vi "Output.vi"(8 "error in (no error)":errorcluster, 11 "Pump Calibration Config in":T1={"Settings"={"Cycle Period"=500.0, "Ismatech"={"VISA resource name"="", "Simulated?"=TRUE, "Pump Number"=1.0, "Reverse?"=FALSE}, "Masterflex"={"VISA resource name"="", "Simulated?"=TRUE, "Pump Number"=1.0, "Reverse?"=FALSE}, "Bronkhorst M13 Settings"={"VISA resource name"="", "Simulated?"=TRUE, "Smoothing Steps"=1}, "PID 2 Parameters"={"Input Device"=enum."Default", "Output Device"=enum."Default"}, "Tacmina Settings"={"Analog DAQ Task"="", "Digital DAQ Task"=""}, "KNF SIMDOS Settings"={"VISA resource name"="", "Simulated?"=TRUE}, "VICI M50 Settings"={"VISA resource name"="", "Pump ID"="", "Pump Head Vol"=0.0, "Reverse?"=FALSE, "Simulated?"=TRUE}, "FLOM Settings"={"VISA resource name"="", "Simulated?"=TRUE, "Pump Number"=0.0}, "Calibration Limits"={"Minimum (ml/min)"=0.0, "Maximum (ml/min)"=0.0, "Steps"=0.0}, "SSI PR Settings"={"VISA resource name"="", "Simulated?"=FALSE}, "Ismatech 4308 Settings"={"VISA resource name"="", "Pump Number"=1, "Channel Number"=0, "Simulated?"=TRUE, "Reverse?"=FALSE}, "Bronkhorst M14 Settings"={"VISA resource name"="", "Simulated?"=FALSE, "Smoothing Steps"=1}}, "Flowmeter Output"=0.0, "Density"=0.0, "FL Temp"=0.0, "Speed %"=0.0, "File Refnum"=refnum, "Pump On?"=enum."Not Initialized"} {"Settings"."Bronkhorst M14 Settings"."Smoothing Steps" min=1 step=1; "Settings"."Ismatech 4308 Settings"."Channel Number" min=0 max=3; "Settings"."Ismatech 4308 Settings"."Pump Number" min=1; "Settings"."Bronkhorst M13 Settings"."Smoothing Steps" min=1 step=1; "Settings"."Masterflex"."Pump Number" min=1.0 max=20.0 step=1.0; "Settings"."Ismatech"."Pump Number" min=1.0 max=20.0 step=1.0}) -> (0 "error out":errorcluster, 3 "Pump Calibration Config Out":T1={"Settings"={"Cycle Period"=500.0, "Ismatech"={"VISA resource name"="", "Simulated?"=TRUE, "Pump Number"=1.0, "Reverse?"=FALSE}, "Masterflex"={"VISA resource name"="", "Simulated?"=TRUE, "Pump Number"=1.0, "Reverse?"=FALSE}, "Bronkhorst M13 Settings"={"VISA resource name"="", "Simulated?"=TRUE, "Smoothing Steps"=1}, "PID 2 Parameters"={"Input Device"=enum."Default", "Output Device"=enum."Default"}, "Tacmina Settings"={"Analog DAQ Task"="", "Digital DAQ Task"=""}, "KNF SIMDOS Settings"={"VISA resource name"="", "Simulated?"=TRUE}, "VICI M50 Settings"={"VISA resource name"="", "Pump ID"="", "Pump Head Vol"=0.0, "Reverse?"=FALSE, "Simulated?"=TRUE}, "FLOM Settings"={"VISA resource name"="", "Simulated?"=TRUE, "Pump Number"=0.0}, "Calibration Limits"={"Minimum (ml/min)"=0.0, "Maximum (ml/min)"=0.0, "Steps"=0.0}, "SSI PR Settings"={"VISA resource name"="", "Simulated?"=FALSE}, "Ismatech 4308 Settings"={"VISA resource name"="", "Pump Number"=1, "Channel Number"=0, "Simulated?"=TRUE, "Reverse?"=FALSE}, "Bronkhorst M14 Settings"={"VISA resource name"="", "Simulated?"=FALSE, "Smoothing Steps"=1}}, "Flowmeter Output"=0.0, "Density"=0.0, "FL Temp"=0.0, "Speed %"=0.0, "File Refnum"=refnum, "Pump On?"=enum."Not Initialized"} {"Settings"."Bronkhorst M14 Settings"."Smoothing Steps" min=1 step=1; "Settings"."Ismatech 4308 Settings"."Channel Number" min=0 max=3; "Settings"."Ismatech 4308 Settings"."Pump Number" min=1; "Settings"."Bronkhorst M13 Settings"."Smoothing Steps" min=1 step=1; "Settings"."Masterflex"."Pump Number" min=1.0 max=20.0 step=1.0; "Settings"."Ismatech"."Pump Number" min=1.0 max=20.0 step=1.0})   [LabVIEW 2018, in "Calibration.lvlib" / "Engine.lvlib"]
uses:
  Engine.lvlib
  Pump Calibration Config.ctl
  Pfizer Timed Seq/Software/Ismatec ISM 831C/Controls/Ismatech ISM831C Settings Cluster.ctl
  Pfizer Timed Seq/Software/Masterflex 7550-30/Controls/Settings Cluster.ctl
  Pfizer Timed Seq/Software/Bronkhorst M13 Flow Meter/Settings Cluster.ctl
  Pfizer Timed Seq/Software/Measure Instrument/PID Input Enum.ctl
  Pfizer Timed Seq/Software/Measure Instrument/PID 2 Output Enum.ctl
  Pfizer Timed Seq/Software/Tacmina QI/Tacmina QI DAQ Setting.ctl
  Pfizer Timed Seq/Software/KNF Pump/Settings Cluster plus SIMDOS.ctl
  Pfizer Timed Seq/Software/VICI M50 Party Mode/Settings Cluster.ctl
  Pfizer Timed Seq/Software/FLOM Pump/Settings Cluster.ctl
  Pfizer Timed Seq/Software/SSI PR Class/SSI PR or LD Settings Cluster.ctl
  Pfizer Timed Seq/Software/Ismatec 78001/Ismatec 4083.ctl
  Pfizer Timed Seq/Software/Bronkhorst M14 Flow Meter/Settings Cluster.ctl
  Pfizer Timed Seq/Software/Ismatec ISM 831C/Ismatec ISM 831C.lvlib
  Pfizer Timed Seq/Software/Masterflex 7550-30/Masterflex 7550-30.lvlib
  Pfizer Timed Seq/Software/VICI M50 Party Mode/VICI M6 M50 Party Mode.lvlib
  Pfizer Timed Seq/Software/Tacmina QI/Tacmina QI.lvlib
  Pfizer Timed Seq/Software/KNF Pump/KNF SIMDOS.lvlib
  Pfizer Timed Seq/Software/FLOM Pump/FLOM Pump.lvlib
  Pfizer Timed Seq/Software/SSI PR Class/SSI PR or LD Pump.lvlib
  Pfizer Timed Seq/Software/Ismatec 78001/Ismatec 4308.lvlib
  Pfizer Timed Seq/Software/Bronkhorst M13 Flow Meter/Bronkhorst M13 Flow Meter.lvlib
  Pfizer Timed Seq/Software/Calibration VIs/Calibration.lvlib
  Pfizer Timed Seq/Software/Bronkhorst M14 Flow Meter/Bronkhorst M14 Flow Meter.lvlib
panel:
  # "Output Instruments"
  # "Input Instruments"
  # "Output Instruments"
  # "Input Instruments"
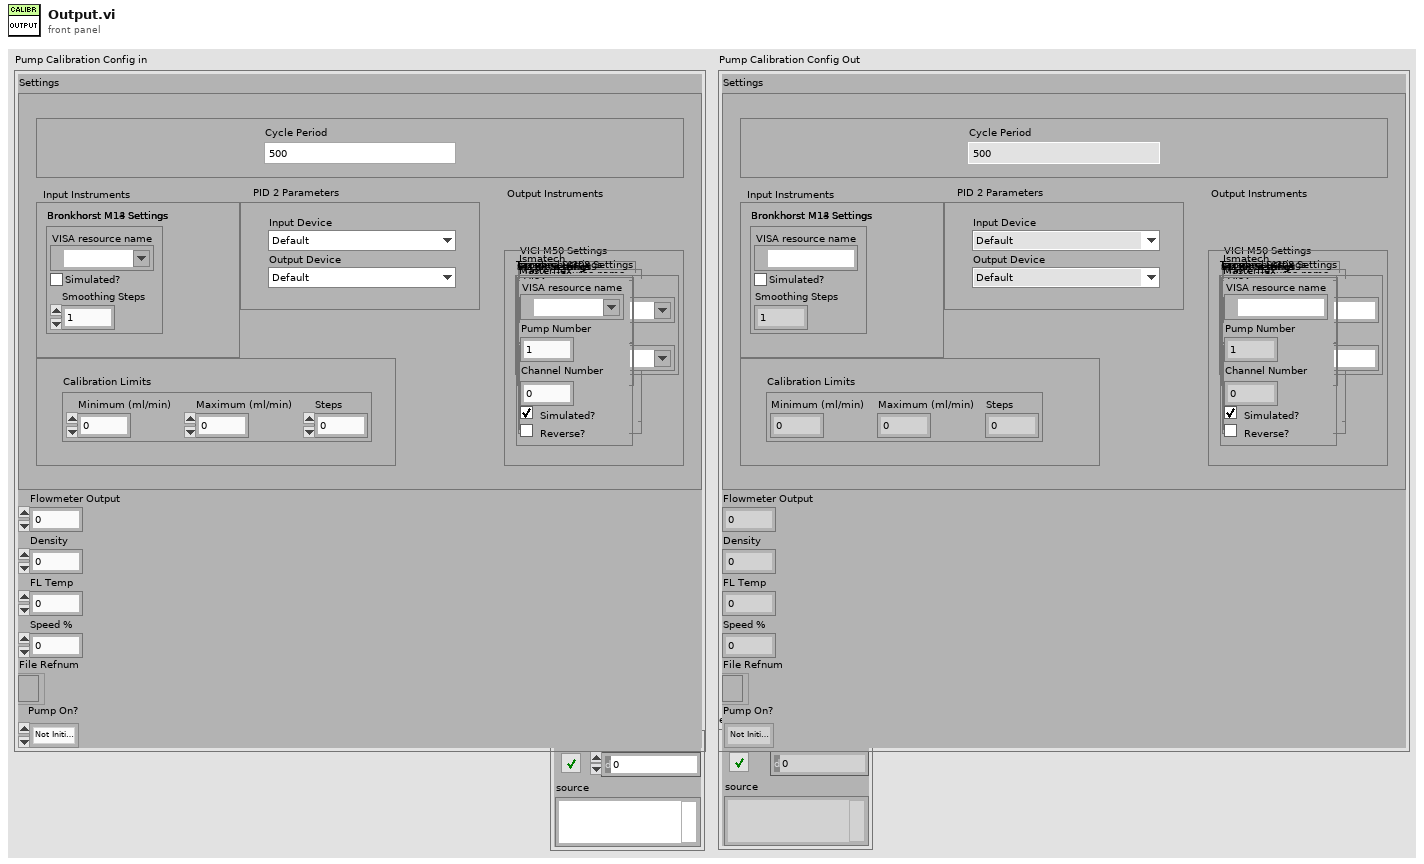
[diagram p1: front panel]
types:
  T1 = typedef "Calibration.lvlib/Pump Calibration Config.ctl" = cluster{"Settings":cluster{"Cycle Period":dbl, "Ismatech":T2, "Masterflex":T3, "Bronkhorst M13 Settings":T4, "PID 2 Parameters":cluster{"Input Device":T5, "Output Device":T6}, "Tacmina Settings":T7, "KNF SIMDOS Settings":T8, "VICI M50 Settings":T9, "FLOM Settings":T10, "Calibration Limits":cluster{"Minimum (ml/min)":dbl, "Maximum (ml/min)":dbl, "Steps":dbl}, "SSI PR Settings":T11, "Ismatech 4308 Settings":T12, "Bronkhorst M14 Settings":T13}, "Flowmeter Output":dbl, "Density":dbl, "FL Temp":dbl, "Speed %":dbl, "File Refnum":refnum<file>, "Pump On?":enum16{"Off", "On", "Not Initialized"}}
  T2 = typedef "Ismatec ISM 831C.lvlib/Ismatech ISM831C Settings Cluster.ctl" = cluster{"VISA resource name":refnum<visa-resource-name>, "Simulated?":bool, "Pump Number":dbl, "Reverse?":bool}
  T3 = typedef "Masterflex 7550-30.lvlib/Settings Cluster.ctl" = cluster{"VISA resource name":refnum<visa-resource-name>, "Simulated?":bool, "Pump Number":dbl, "Reverse?":bool}
  T4 = typedef "Bronkhorst M13 Flow Meter.lvlib/Settings Cluster.ctl" = cluster{"VISA resource name":refnum<visa-resource-name>, "Simulated?":bool, "Smoothing Steps":i32}
  T5 = typedef "PID Input Enum.ctl" = enum16{"Default", "Bronkhorst M13", "Bronkhorst M14", "Scale Rate of Change"}
  T6 = typedef "PID 2 Output Enum.ctl" = enum16{"Default", "Ismatec ISM 4308", "Ismatec ISM 831C", "Masterflex 7550-30", "VICI M6", "VICI M50", "Tacmina QI", "KNF SIMDOS", "ASIA Type C", "FLOM UI-22-11", "SSI PR/LD", "SSI P40", "Masterflex 75211-70"}
  T7 = typedef "Tacmina QI.lvlib/Tacmina QI DAQ Setting.ctl" = cluster{"Analog DAQ Task":refnum<k21>, "Digital DAQ Task":refnum<k21>}
  T8 = typedef "KNF SIMDOS.lvlib/Settings Cluster plus SIMDOS.ctl" = cluster{"VISA resource name":refnum<visa-resource-name>, "Simulated?":bool}
  T9 = typedef "VICI M6 M50 Party Mode.lvlib/Settings Cluster.ctl" = cluster{"VISA resource name":refnum<visa-resource-name>, "Pump ID":string, "Pump Head Vol":dbl, "Reverse?":bool, "Simulated?":bool}
  T10 = typedef "FLOM Pump.lvlib/Settings Cluster.ctl" = cluster{"VISA resource name":refnum<visa-resource-name>, "Simulated?":bool, "Pump Number":dbl}
  T11 = typedef "SSI PR or LD Pump.lvlib/SSI PR or LD Settings Cluster.ctl" = cluster{"VISA resource name":refnum<visa-resource-name>, "Simulated?":bool}
  T12 = typedef "Ismatec 4308.lvlib/Ismatec 4083.ctl" = cluster{"VISA resource name":refnum<visa-resource-name>, "Pump Number":i16, "Channel Number":i16, "Simulated?":bool, "Reverse?":bool}
  T13 = typedef "Bronkhorst M14 Flow Meter.lvlib/Settings Cluster.ctl" = cluster{"VISA resource name":refnum<visa-resource-name>, "Simulated?":bool, "Smoothing Steps":i32}
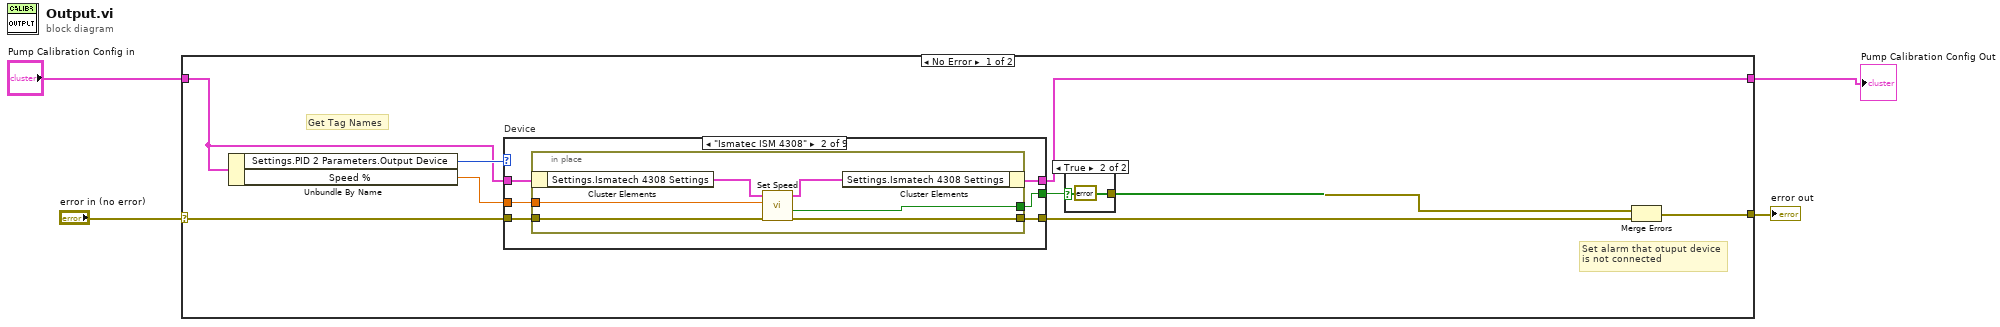
[diagram p0: block diagram]
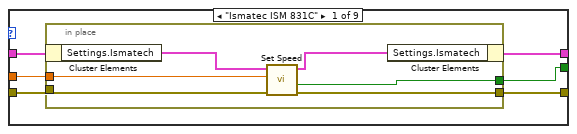
[diagram p2: hidden frame]
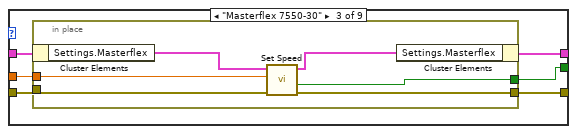
[diagram p3: hidden frame]
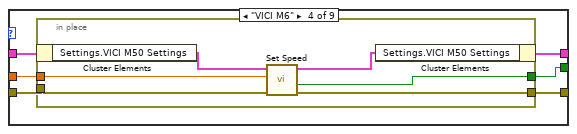
[diagram p4: hidden frame]
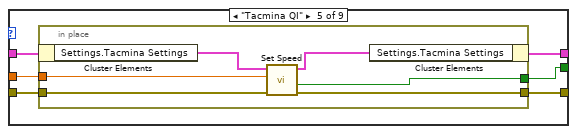
[diagram p5: hidden frame]
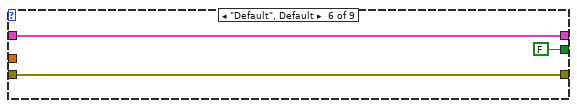
[diagram p6: hidden frame]
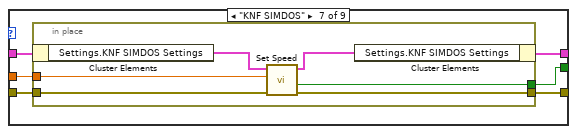
[diagram p7: hidden frame]
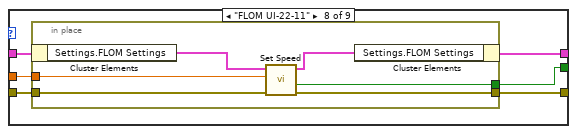
[diagram p8: hidden frame]
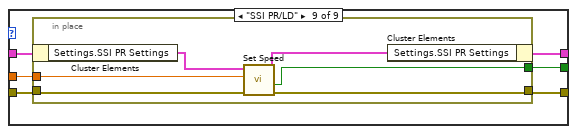
[diagram p9: hidden frame]
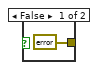
[diagram p10: hidden frame]
diagram:
  n1 = case shown="No Error" "error in (no error)" {
    selector: "error in (no error)" -> [w11 w116]
    tunnel: [w7 w116] -> w3
    tunnel: "Pump Calibration Config in" -> [w9 w115]
    tunnel: [w10 w115] -> w2
    frame No Error {
      # "Get Tag Names"
      # "Set alarm that otuput device\nis not connected"
      n2 = Unbundle By Name(w9) -> ("Settings.PID 2 Parameters.Output Device"=w13:T6, "Speed %"=w12:dbl)
      n3 = case "Device" shown="\"Ismatec ISM 4308\"" w13 {
        tunnel: w12 -> [w17 w26 w41 w55 w67 _ w82 w93 w106]
        tunnel: w11 -> [w19 w31 w43 w54 w66 w75 w81 w94 w105]
        tunnel: [w18 w27 w42 w53 w65 w75 w80 w91 w104] -> w6
        tunnel: w9 -> [w15 w30 w39 w51 w63 w76 w78 w90 w102]
        tunnel: [w14 w29 w38 w50 w62 w76 w77 w89 w101] -> w10
        tunnel: [w16 w28 w40 w52 w64 FALSE ("Connection Error") w79 w92 w103] -> w8
        frame "Ismatec ISM 831C" {
          n4 = in-place {
            in-place-border: w19 -> [w25]
            in-place-border: [w24] -> w18
            in-place-border: w17 -> [w23]
            in-place-border: [w22] -> w16
            n5 = in-place-cluster #1(w15) -> ("Settings.Ismatech"=w21:T2)
            n6 = call "Set Speed.vi"("error in (no error)"=w25, "Speed (%)"=w23, "Ismatech Settings In"=w21) -> ("error out"=w24:errorcluster, "Connection Error"=w22:bool, "Ismatech Settings Out"=w20:T2)  [unwired: 6 in]
            n7 = in-place-cluster #1("Settings.Ismatech"=w20) -> (w14:T1)
          }
        }
        frame "Ismatec ISM 4308" {
          n8 = in-place {
            in-place-border: w31 -> [w34]
            in-place-border: [w35] -> w27
            in-place-border: w26 -> [w33]
            in-place-border: [w32] -> w28
            n9 = in-place-cluster #2(w30) -> ("Settings.Ismatech 4308 Settings"=w37:T12)
            n10 = call "Set Speed.vi"("error in (no error)"=w34, "Speed (%)"=w33, "Ismatech 3 Channel Settings In"=w37) -> ("error out"=w35:errorcluster, "Connection Error"=w32:bool, "Ismatech 3 Channel Settings Out"=w36:T12)  [unwired: 5 in, 1 out]
            n11 = in-place-cluster #2("Settings.Ismatech 4308 Settings"=w36) -> (w29:T1)
          }
        }
        frame "Masterflex 7550-30" {
          n12 = in-place {
            in-place-border: w43 -> [w49]
            in-place-border: [w48] -> w42
            in-place-border: w41 -> [w47]
            in-place-border: [w46] -> w40
            n13 = in-place-cluster #3(w39) -> ("Settings.Masterflex"=w45:T3)
            n14 = call "Set Speed.vi"("error in (no error)"=w49, "speed"=w47, "Masterflex Settings in"=w45) -> ("error out"=w48:errorcluster, "Connection Error"=w46:bool, "Masterflex Settings out"=w44:T3)  [unwired: 6 in]
            n15 = in-place-cluster #3("Settings.Masterflex"=w44) -> (w38:T1)
          }
        }
        frame "VICI M6" {
          n16 = in-place {
            in-place-border: w55 -> [w61]
            in-place-border: w54 -> [w60]
            in-place-border: [w59] -> w53
            in-place-border: [w58] -> w52
            n17 = in-place-cluster #4(w51) -> ("Settings.VICI M50 Settings"=w56:T9)
            n18 = call "Set Speed.vi"("error in (no error)"=w60, "Flow Rate (mL/min)"=w61, "VICI Settings In"=w56) -> ("error out"=w59:errorcluster, "Connection Error"=w58:bool, "VICI Settings Out"=w57:T9)  [unwired: 6 in]
            n19 = in-place-cluster #4("Settings.VICI M50 Settings"=w57) -> (w50:T1)
          }
        }
        frame "Tacmina QI" {
          n20 = in-place {
            in-place-border: w67 -> [w73]
            in-place-border: w66 -> [w72]
            in-place-border: [w71] -> w65
            in-place-border: [w70] -> w64
            n21 = in-place-cluster #5(w63) -> ("Settings.Tacmina Settings"=w68:T7)
            n22 = call "Set Speed.vi"("error in"=w72, "Pump %"=w73, "Tacmina Settings in"=w68) -> ("error out"=w71:errorcluster, "Connection Error"=w70:bool, "Tacmina Settings out"=w69:T7)  [unwired: 6 in]
            n23 = in-place-cluster #5("Settings.Tacmina Settings"=w69) -> (w62:T1)
          }
        }
        frame "Default", Default {
        }
        frame "KNF SIMDOS" {
          n24 = in-place {
            in-place-border: w82 -> [w88]
            in-place-border: w81 -> [w87]
            in-place-border: [w86] -> w80
            in-place-border: [w85] -> w79
            n25 = in-place-cluster #6(w78) -> ("Settings.KNF SIMDOS Settings"=w84:T8)
            n26 = call "Set Speed.vi"("error in (no error)"=w87, "FlowRate"=w88, "KNF Settings In"=w84) -> ("error out"=w86:errorcluster, "Connection Error"=w85:bool, "KNF Settings Out"=w83:T8)  [unwired: 6 in]
            n27 = in-place-cluster #6("Settings.KNF SIMDOS Settings"=w83) -> (w77:T1)
          }
        }
        frame "FLOM UI-22-11" {
          n28 = in-place {
            in-place-border: w94 -> [w100]
            in-place-border: w93 -> [w99]
            in-place-border: [w98] -> w92
            in-place-border: [w97] -> w91
            n29 = in-place-cluster #7(w90) -> ("Settings.FLOM Settings"=w96:T10)
            n30 = call "Set Speed.vi"("error in (no error)"=w100, "speed"=w99, "FLOM Settings in"=w96) -> ("error out"=w97:errorcluster, "Connection Error"=w98:bool, "FLOM Settings out"=w95:T10)  [unwired: 6 in]
            n31 = in-place-cluster #7("Settings.FLOM Settings"=w95) -> (w89:T1)
          }
        }
        frame "SSI PR/LD" {
          n32 = in-place {
            in-place-border: w106 -> [w112]
            in-place-border: w105 -> [w111]
            in-place-border: [w110] -> w104
            in-place-border: [w109] -> w103
            n33 = in-place-cluster #8(w102) -> ("Settings.SSI PR Settings"=w108:T11)
            n34 = call "Set Speed.vi"("error in (no error)"=w111, "speed (ml/min)"=w112, "SSI PR Settings In"=w108) -> ("error out"=w110:errorcluster, "Connection Error"=w109:bool, "SSI PR Settings Out"=w107:T11)  [unwired: 6 in]
            n35 = in-place-cluster #8("Settings.SSI PR Settings"=w107) -> (w101:T1)
          }
        }
      }
      n36 = case shown="True" w8 {
        tunnel: [errorcluster {"status"=FALSE, "code"=0, "source"=""} ("error constant") errorcluster {"status"=TRUE, "code"=2, "source"="Output Error"} ("error constant")] -> w5
        frame False {
        }
        frame True {
        }
      }
      n37 = Merge Errors(w5, w6) -> (w7:errorcluster)
    }
    frame Error {
    }
  }
  "error out" <- w3
  "Pump Calibration Config Out" <- w2
